vi "Get BLISS_Select Random Image.vi"(7 "BLISS Type":enum16{"Reject Images", "PBQA Images"}(ring), 8 "error in":errorcluster, 11 "Data Parameters in":T1={"Start Time"=timestamp(3690155740.033191 s since 1904-01-01), "Save to Folder"=path "", "Forces in Theater"=[{"Force Commander"="BlissUT124", "Units"=[]}, {"Force Commander"="BlissMP146", "Units"=[]}, {"Force Commander"="BlissMP145", "Units"=[]}, {"Force Commander"="BlissMP140", "Units"=[]}, {"Force Commander"="BlissMP137", "Units"=[]}, {"Force Commander"="BlissMP135", "Units"=[]}, {"Force Commander"="BlissMP134", "Units"=[]}, {"Force Commander"="BlissMP132", "Units"=[]}, {"Force Commander"="BlissMA109", "Units"=[]}, {"Force Commander"="BlissMA107", "Units"=[]}, {"Force Commander"="BlissMA106", "Units"=[]}, {"Force Commander"="BlissMA101", "Units"=[]}, {"Force Commander"="BlissLU118", "Units"=[]}, {"Force Commander"="BlissLU117", "Units"=[]}, {"Force Commander"="BlissLU116", "Units"=[]}, {"Force Commander"="BlissLU115", "Units"=[]}, {"Force Commander"="BlissLU114", "Units"=[]}, {"Force Commander"="BlissLU113", "Units"=[]}, {"Force Commander"="BlissLU111", "Units"=[]}, {"Force Commander"="BlissLL185", "Units"=[]}, {"Force Commander"="BlissLL183", "Units"=[]}, {"Force Commander"="BlissLL173", "Units"=[]}, {"Force Commander"="BlissLL172", "Units"=[]}, {"Force Commander"="BlissLL171", "Units"=[]}, {"Force Commander"="BlissJH103", "Units"=[]}, {"Force Commander"="BlissJH102", "Units"=[]}, {"Force Commander"="BlissJH101", "Units"=[]}, {"Force Commander"="BlissJE116", "Units"=[]}, {"Force Commander"="BlissJE115", "Units"=[]}, {"Force Commander"="BlissJE114", "Units"=[]}, {"Force Commander"="BlissJE111", "Units"=[]}, {"Force Commander"="BlissHD183", "Units"=[]}, {"Force Commander"="BlissHD182", "Units"=[]}, {"Force Commander"="BlissHD181", "Units"=[]}, {"Force Commander"="BlissGPDFFPL", "Units"=[]}, {"Force Commander"="BlissEUWIPES", "Units"=[]}, {"Force Commander"="BlissEU179", "Units"=[]}, {"Force Commander"="BlissEU178", "Units"=[]}, {"Force Commander"="BlissEU177", "Units"=[]}, {"Force Commander"="Blissdvds02", "Units"=[]}, {"Force Commander"="BlissDOWIPES", "Units"=[]}, {"Force Commander"="BlissCR022", "Units"=[]}, {"Force Commander"="BlissCR021", "Units"=[]}, {"Force Commander"="BlissCG167", "Units"=[]}, {"Force Commander"="BlissCG166", "Units"=[]}, {"Force Commander"="BlissCG161", "Units"=[]}, {"Force Commander"="BlissCG160", "Units"=[]}, {"Force Commander"="BlissCG159", "Units"=[]}, {"Force Commander"="BlissCG158", "Units"=[]}, {"Force Commander"="BlissCG157", "Units"=[]}, {"Force Commander"="BlissCG156", "Units"=[]}, {"Force Commander"="BlissCG151", "Units"=[]}, {"Force Commander"="BlissCB172", "Units"=[]}, {"Force Commander"="BlissCB171", "Units"=[]}, {"Force Commander"="BlissCB108", "Units"=[]}, {"Force Commander"="BlissCB107", "Units"=[]}, {"Force Commander"="BlissBV181", "Units"=[]}, {"Force Commander"="BlissBV162", "Units"=[]}, {"Force Commander"="BlissAK177", "Units"=[]}, {"Force Commander"="BlissAK176", "Units"=[]}, {"Force Commander"="BlissAK175", "Units"=[]}, {"Force Commander"="BlissAK174", "Units"=[]}, {"Force Commander"="BlissAK173", "Units"=[]}, {"Force Commander"="BlissAK172", "Units"=[]}, {"Force Commander"="BlissAK171", "Units"=[]}, {"Force Commander"="BlissAK139", "Units"=[]}, {"Force Commander"="BlissAK134", "Units"=[]}, {"Force Commander"="BlissAK131", "Units"=[]}, {"Force Commander"="BlissAH163", "Units"=[]}, {"Force Commander"="BlissAH162", "Units"=[]}, {"Force Commander"="BlissAH161", "Units"=[]}, {"Force Commander"="BlissAH122", "Units"=[]}, {"Force Commander"="BlissAH121", "Units"=[]}, {"Force Commander"="BlissAD106", "Units"=[]}, {"Force Commander"="BlissAD104", "Units"=[]}, {"Force Commander"="BlissAB105", "Units"=[]}, {"Force Commander"="BlissAB104", "Units"=[]}]}) -> (0 "error out":errorcluster, 3 "Data Parameters out":T1={"Start Time"=timestamp(3690155740.033191 s since 1904-01-01), "Save to Folder"=path "D:/One Drive PG/Procter and Gamble/Varghese, Jacob - Deep Learning Vision System/Front Ear Foldover/BLISS Rejects (only R325 + R326) - not reviewed", "Forces in Theater"=[{"Force Commander"="BlissUT124", "Units"=[]}, {"Force Commander"="BlissMP146", "Units"=[]}, {"Force Commander"="BlissMP145", "Units"=[]}, {"Force Commander"="BlissMP140", "Units"=[]}, {"Force Commander"="BlissMP137", "Units"=[]}, {"Force Commander"="BlissMP135", "Units"=[]}, {"Force Commander"="BlissMP134", "Units"=[]}, {"Force Commander"="BlissMP132", "Units"=[]}, {"Force Commander"="BlissMA109", "Units"=[]}, {"Force Commander"="BlissMA107", "Units"=[]}, {"Force Commander"="BlissMA106", "Units"=[]}, {"Force Commander"="BlissMA101", "Units"=[]}, {"Force Commander"="BlissLU118", "Units"=[]}, {"Force Commander"="BlissLU117", "Units"=[]}, {"Force Commander"="BlissLU116", "Units"=[]}, {"Force Commander"="BlissLU115", "Units"=[]}, {"Force Commander"="BlissLU114", "Units"=[]}, {"Force Commander"="BlissLU113", "Units"=[]}, {"Force Commander"="BlissLU111", "Units"=[]}, {"Force Commander"="BlissLL185", "Units"=[]}, {"Force Commander"="BlissLL183", "Units"=[]}, {"Force Commander"="BlissLL173", "Units"=[]}, {"Force Commander"="BlissLL172", "Units"=[]}, {"Force Commander"="BlissLL171", "Units"=[]}, {"Force Commander"="BlissJH103", "Units"=[]}, {"Force Commander"="BlissJH102", "Units"=[]}, {"Force Commander"="BlissJH101", "Units"=[]}, {"Force Commander"="BlissJE116", "Units"=[]}, {"Force Commander"="BlissJE115", "Units"=[]}, {"Force Commander"="BlissJE114", "Units"=[]}, {"Force Commander"="BlissJE111", "Units"=[]}, {"Force Commander"="BlissHD183", "Units"=[]}, {"Force Commander"="BlissHD182", "Units"=[]}, {"Force Commander"="BlissHD181", "Units"=[]}, {"Force Commander"="BlissGPDFFPL", "Units"=[]}, {"Force Commander"="BlissEUWIPES", "Units"=[]}, {"Force Commander"="BlissEU179", "Units"=[]}, {"Force Commander"="BlissEU178", "Units"=[]}, {"Force Commander"="BlissEU177", "Units"=[]}, {"Force Commander"="Blissdvds02", "Units"=[]}, {"Force Commander"="BlissDOWIPES", "Units"=[]}, {"Force Commander"="BlissCR022", "Units"=[]}, {"Force Commander"="BlissCR021", "Units"=[]}, {"Force Commander"="BlissCG167", "Units"=[]}, {"Force Commander"="BlissCG166", "Units"=[]}, {"Force Commander"="BlissCG161", "Units"=[]}, {"Force Commander"="BlissCG160", "Units"=[]}, {"Force Commander"="BlissCG159", "Units"=[]}, {"Force Commander"="BlissCG158", "Units"=[]}, {"Force Commander"="BlissCG157", "Units"=[]}, {"Force Commander"="BlissCG156", "Units"=[]}, {"Force Commander"="BlissCG151", "Units"=[]}, {"Force Commander"="BlissCB172", "Units"=[]}, {"Force Commander"="BlissCB171", "Units"=[]}, {"Force Commander"="BlissCB108", "Units"=[]}, {"Force Commander"="BlissCB107", "Units"=[]}, {"Force Commander"="BlissBV181", "Units"=[]}, {"Force Commander"="BlissBV162", "Units"=[]}, {"Force Commander"="BlissAK177", "Units"=[]}, {"Force Commander"="BlissAK176", "Units"=[]}, {"Force Commander"="BlissAK175", "Units"=[]}, {"Force Commander"="BlissAK174", "Units"=[]}, {"Force Commander"="BlissAK173", "Units"=[]}, {"Force Commander"="BlissAK172", "Units"=[]}, {"Force Commander"="BlissAK171", "Units"=[]}, {"Force Commander"="BlissAK139", "Units"=[]}, {"Force Commander"="BlissAK134", "Units"=[]}, {"Force Commander"="BlissAK131", "Units"=[]}, {"Force Commander"="BlissAH163", "Units"=[]}, {"Force Commander"="BlissAH162", "Units"=[]}, {"Force Commander"="BlissAH161", "Units"=[]}, {"Force Commander"="BlissAH122", "Units"=[]}, {"Force Commander"="BlissAH121", "Units"=[]}, {"Force Commander"="BlissAD106", "Units"=[]}, {"Force Commander"="BlissAD104", "Units"=[]}, {"Force Commander"="BlissAB105", "Units"=[]}, {"Force Commander"="BlissAB104", "Units"=[]}]})   [LabVIEW 2020]
uses:
  MC5e Gobal_Variables.vi
  Get BLISS_Data Paramter Actions.ctl
  MC5e Squad_Info.ctl
  MC5e Unit_Status_List.ctl
  MC5e Data_Parameters.ctl
  MC5e Terrain types.ctl
  Location.ctl
  MC5e Unit.ctl
  MC5e Force.ctl
panel:
  out "Aborting":bool
  in  "Tab Control":enum32{"PBQA", "Reject"}(tab)
  out "PBQA File List":string[](array[string])
  out "Reject File List":string[](array[string])
  out "Processing":bool=TRUE
  in  "Abort Process Button":bool
  out "Searching for":enum16{"Reject Images", "PBQA Images"}(ring)
  out "Server Name":string
  out "Reject Date":string
  out "Reject View":string
  out "Reject Code":string
  out "PBQA View":string
  out "PBQA Size":string
  out "PBQA date":string
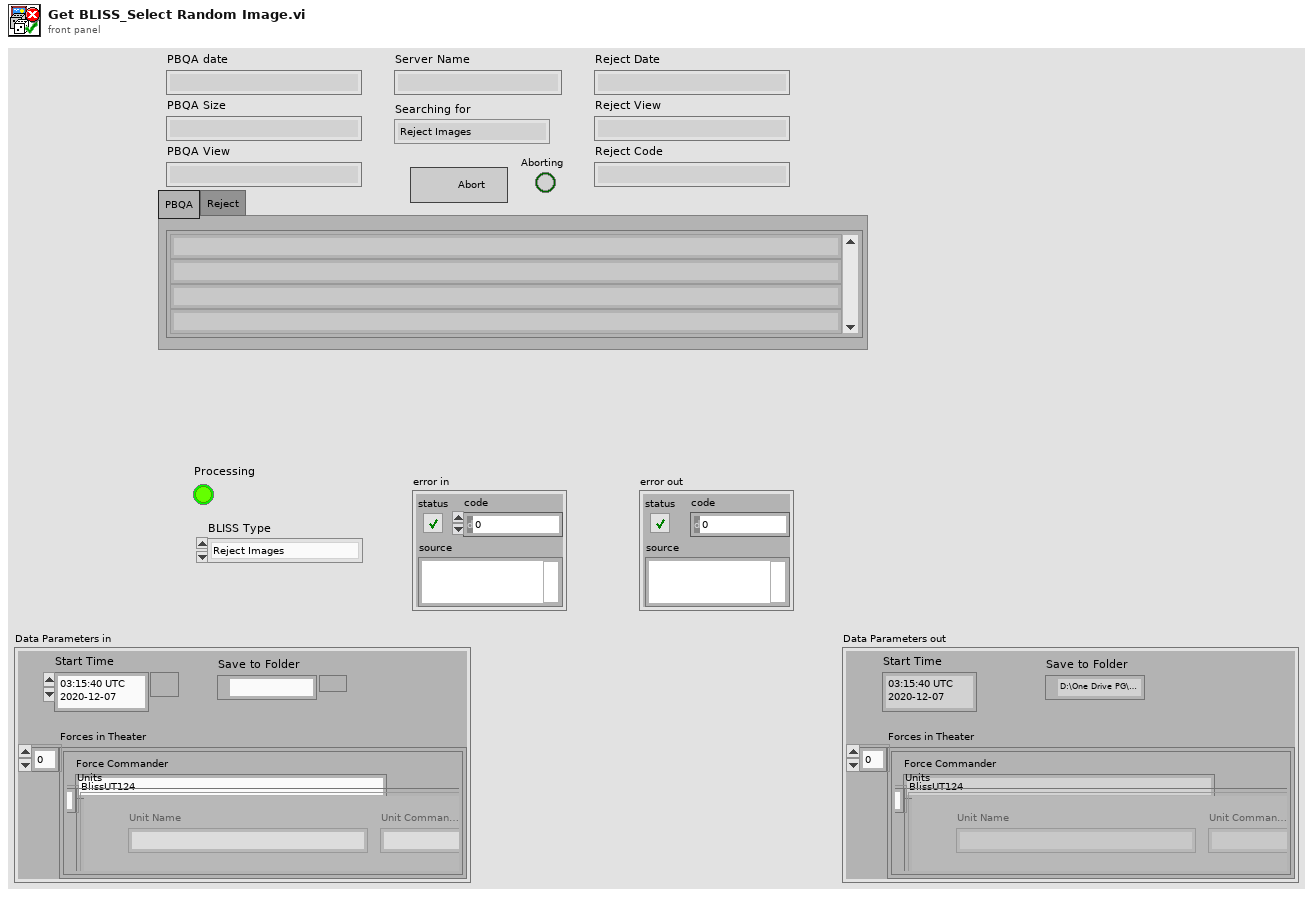
[diagram p1: front panel]
types:
  T1 = typedef "MC5e Data_Parameters.ctl" = cluster{"Start Time":timestamp, "Save to Folder":path, "Forces in Theater":T2[]}
  T2 = typedef "MC5e Force.ctl" = cluster{"Force Commander":string, "Units":T3[]}
  T3 = typedef "MC5e Unit.ctl" = cluster{"Squad List":T4, "Unit Fatigue Level":enum16{"Not Fatigued", "Fatigued", "Seriously Fatigued"}, "Flying Unit":bool, "Mounted Unit":bool, "Difficult Terrain Types":T6, "Full BR":dbl, "Defending from Stronghold":bool, "Speed":dbl, "Capacity %":dbl, "Morale":dbl, "Current BR":dbl, "Location":T7, "Unit Name":string, "Unit Commander":string, "Unit Notes":string}
  T4 = typedef "MC5e Unit_Status_List.ctl" = T5[]
  T5 = typedef "MC5e Squad_Info.ctl" = cluster{"Squad Name":string, "# Soldiers":dbl, "Battle Rating":dbl, "Flying":bool, "Mounted":bool, "Speed":dbl, "Range":dbl, "Morale":dbl, "Token Image":variant, "Max Endurance":dbl, "Current Endurance":dbl, "Difficult Terrain":T6}
  T6 = typedef "MC5e Terrain types.ctl" = cluster{"Artic / snow / ice)":bool, "Coast":bool, "Desert / sand":bool, "Forest / woodland":bool, "Grassland / plains":bool, "Mountain / canyons":bool, "Underdark / caverns":bool, "Acquatic / rivers, lakes, ocean":bool}
  T7 = typedef "Location.ctl" = cluster{"X coordinate":dbl, "Y coordinate":dbl}
  T8 = typedef "Get BLISS_Data Paramter Actions.ctl" = enum16{"Initialize", "Increment Index", "Reset Results", "Update", "Read"}
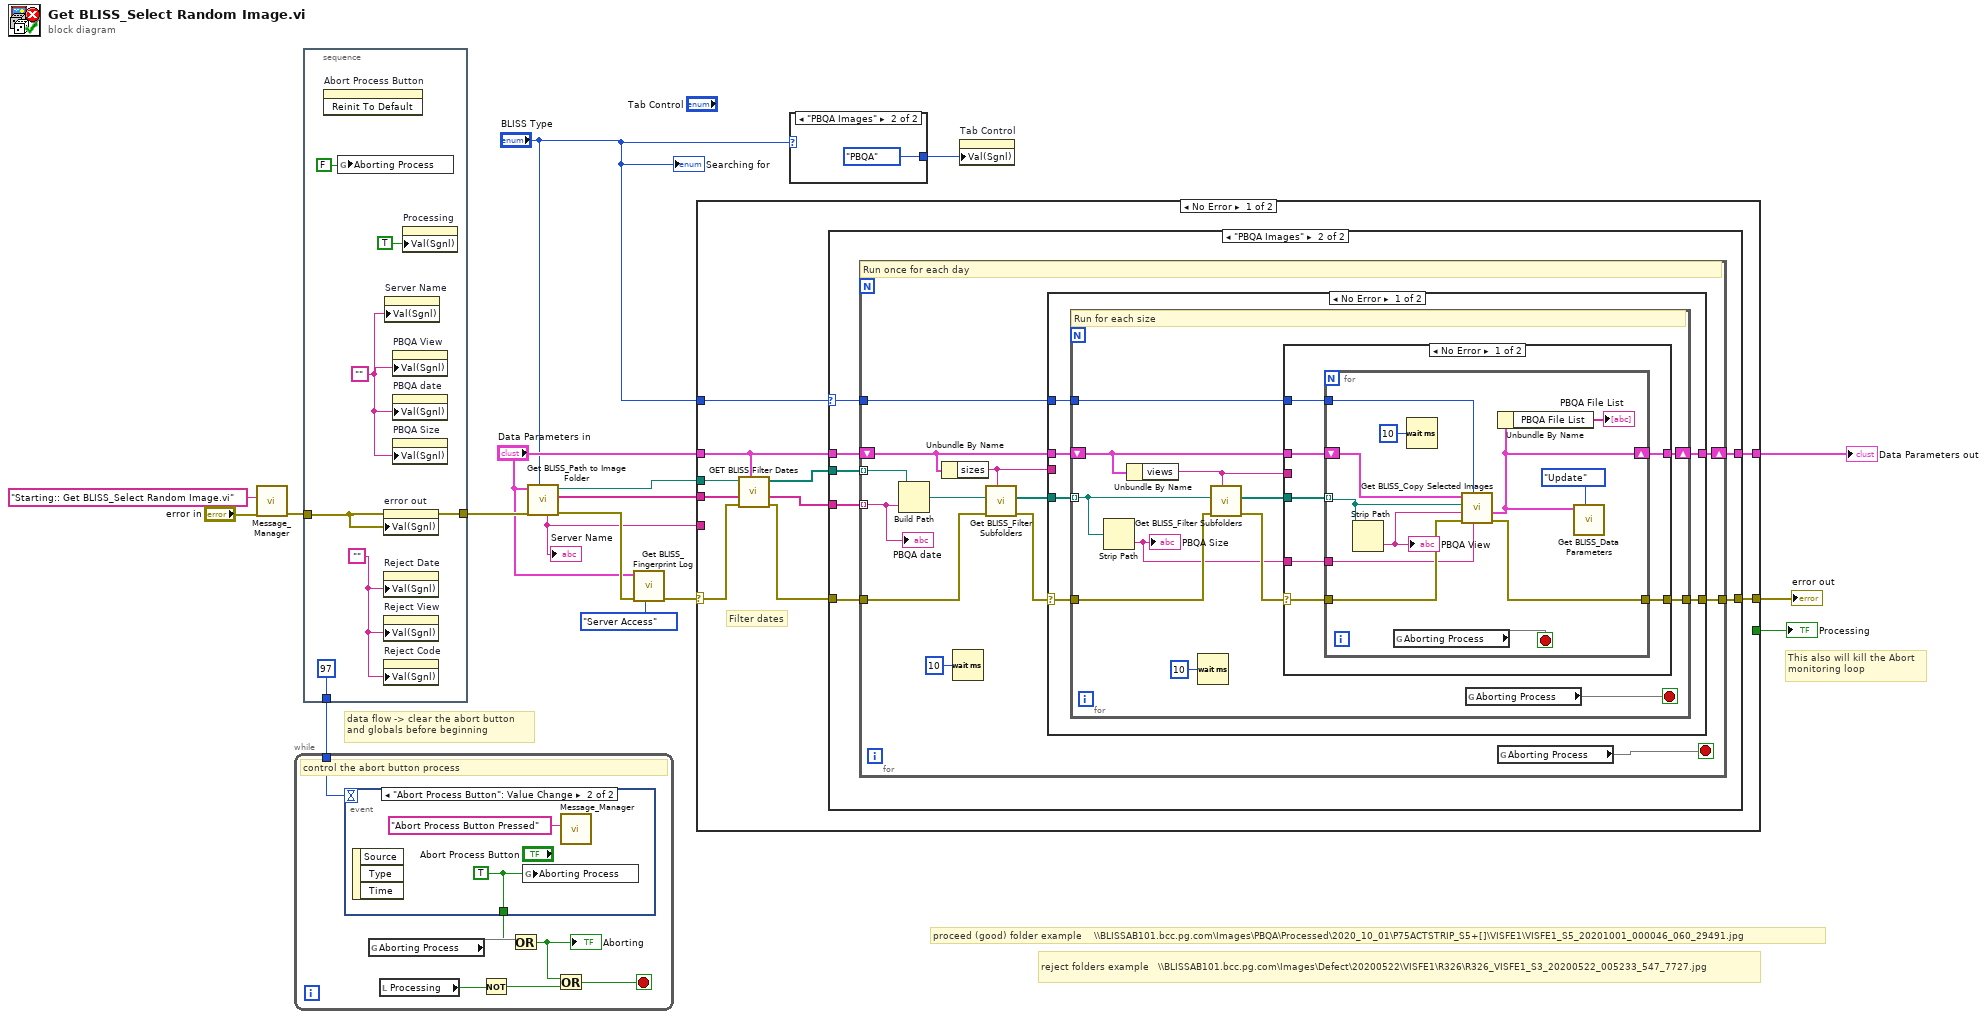
[diagram p0: block diagram]
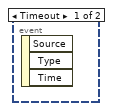
[diagram p2: hidden frame]
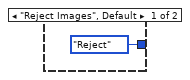
[diagram p3: hidden frame]
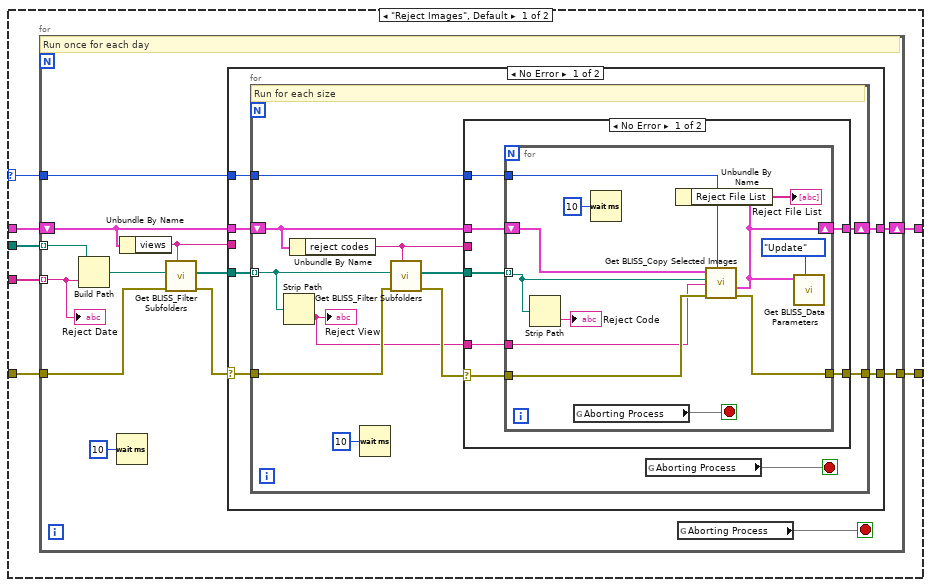
[diagram p4: hidden frame]
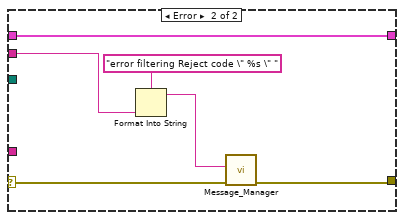
[diagram p5: hidden frame]
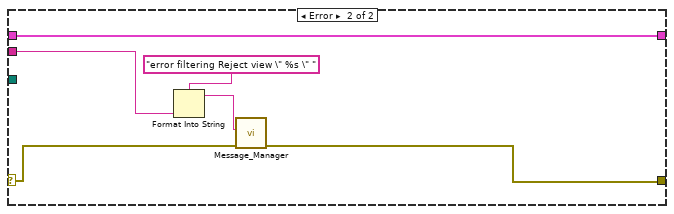
[diagram p6: hidden frame]
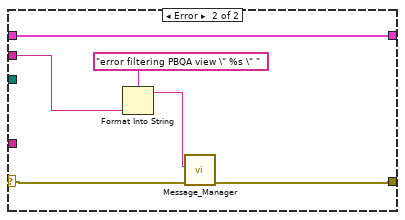
[diagram p7: hidden frame]
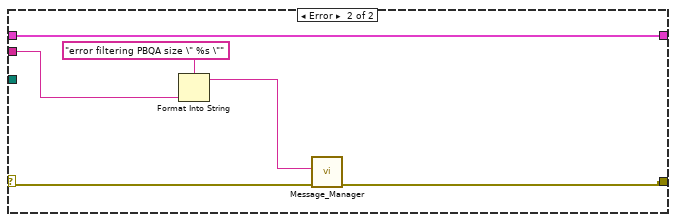
[diagram p8: hidden frame]
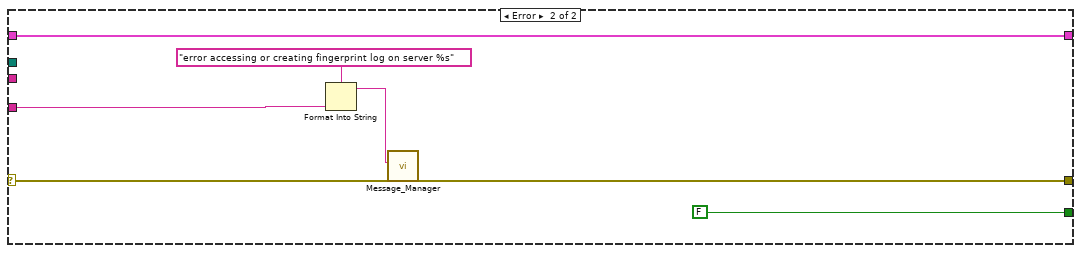
[diagram p9: hidden frame]
diagram:
  # "This also will kill the Abort\nmonitoring loop"
  # "data flow -> clear the abort button \nand globals before beginning"
  # "reject folders example   \\\\BLISSAB101.bcc.pg.com\\Images\\Defect\\20200522\\VISFE1\\R326\\R326_VISFE1_S3_20200522_005233_547_7727.jpg"
  # "proceed (good) folder example    \\\\BLISSAB101.bcc.pg.com\\Images\\PBQA\\Processed\\2020_10_01\\P75ACTSTRIP_S5+[]\\VISFE1\\VISFE1_S5_20201001_000046_060_29491.jpg"
  n1 = call "Message_Manager.vi"("error in"="error in", "New Entry"="Starting:: Get BLISS_Select Random Image.vi") -> ("error out"=w10:errorcluster)  [unwired: 4 in, 5 out]
  n2 = stacked-sequence {
    tunnel: w10 -> [w23]
    tunnel: [w22] -> w13
    tunnel: [u32 97] -> w2
    frame #0 {
      w21 = ""
      w19 = ""
      n3 = invoke on="Abort Process Button" class="Bool" method="Reinit To Default"() -> ()  [unwired: 3 in, 3 out]
      n4 = global write "MC5e Gobal_Variables.vi" "Aborting Process"(FALSE ("Value (Signaling)")) -> ()
      n5 = property on="error out" class="Clust (strict)"(error in=w23, "Val(Sgnl)"=w23) -> (error out=w22:errorcluster)  [unwired: 1 in, 1 out]
      n6 = property on="Reject Date" class="Str"("Val(Sgnl)"=w21) -> ()  [unwired: 2 in, 2 out]
      n7 = property on="Reject View" class="Str"("Val(Sgnl)"=w21) -> ()  [unwired: 2 in, 2 out]
      n8 = property on="Reject Code" class="Str"("Val(Sgnl)"=w21) -> ()  [unwired: 2 in, 2 out]
      n9 = property on="Server Name" class="Str"("Val(Sgnl)"=w19) -> ()  [unwired: 2 in, 2 out]
      n10 = property on="PBQA View" class="Str"("Val(Sgnl)"=w19) -> ()  [unwired: 2 in, 2 out]
      n11 = property on="PBQA date" class="Str"("Val(Sgnl)"=w19) -> ()  [unwired: 2 in, 2 out]
      n12 = property on="PBQA Size" class="Str"("Val(Sgnl)"=w19) -> ()  [unwired: 2 in, 2 out]
      n13 = property on="Processing" class="Bool (strict)"("Val(Sgnl)"=TRUE ("Value (Signaling)")) -> ()  [unwired: 2 in, 2 out]
    }
  }
  n14 = while {
    tunnel: w2 -> [w28]
    stop <- w29 stop-if-true
    # "control the abort button process"
    n15 = event shown="[1] \"Abort Process Button\": Value Change" {
      selector: _ -> [_ _]
      dyn-events: _ -> [_ _]
      timeout: w28 -> [_ _]
      tunnel: [_ w32] -> w26
      event Timeout {
        n16 = event-data() -> ()  [unwired: 1 in, 3 out]
      }
      event "Abort Process Button": Value Change {
        w32 = TRUE ("Aborting Process")
        n17 = event-data() -> ()  [unwired: 1 in, 3 out]
        n18 = global write "MC5e Gobal_Variables.vi" "Aborting Process"(w32) -> ()
        n19 = call "Message_Manager.vi"("New Entry"="Abort Process Button Pressed") -> ()  [unwired: 5 in, 6 out]
      }
    }
    n20 = global read "MC5e Gobal_Variables.vi" "Aborting Process"() -> (w27)
    n21 = local read "Processing"() -> (w31:bool)
    n22 = Not(x=w31) -> (.not. x?=w30:bool)
    n23 = Or(x=w26, y=w27) -> (x .or. y?=w25:bool)
    "Aborting" <- w25
    n24 = Or(x=w25, y=w30) -> (x .or. y?=w29:bool)
  }
  n25 = call "Get BLISS_Path to Image Folder.vi"("BLISS Type"="BLISS Type", "error in (no error)"=w13, "Data Parameters in"="Data Parameters in") -> ("error out"=w8:errorcluster, "Dates (folders)"=w16:string[], "Server Images Path"=w17:path, "Server Name"=w7:string)  [unwired: 5 in]
  "Server Name" <- w7
  n26 = call "Get BLISS_Fingerprint Log.vi"("Action"=enum16{"Server Access", "File Access"}."Server Access", "error in (no error)"=w8, "Data Parameters in"="Data Parameters in") -> ("error out"=w1:errorcluster)  [unwired: 8 in]
  n27 = case shown="No Error" w1 {
    selector: w1 -> [w37 w187]
    tunnel: w16 -> [w39 _]
    tunnel: w17 -> [w40 _]
    tunnel: [w43 w187] -> w15
    tunnel: "Data Parameters in" -> [w34 w186]
    tunnel: [w42 w186] -> w9
    tunnel: "BLISS Type" -> [w41 _]
    tunnel: [_ FALSE] -> w14
    tunnel: w7 -> [_ w182]
    frame No Error {
      # "Filter dates"
      n28 = call "GET BLISS Filter Dates.vi"("Data Parameters in"=w34, "error in"=w37, "Dates (folders)"=w39, "Server Images Path"=w40) -> ("error out"=w36:errorcluster, "Valid Dates"=w35:string[], "Valid Paths"=w38:path[])  [unwired: 5 in]
      n29 = case shown="\"PBQA Images\"" w41 {
        selector: w41 -> [w44 w113]
        tunnel: w38 -> [w50 w119]
        tunnel: w35 -> [w49 w118]
        tunnel: [w48 w117] -> w43
        tunnel: w34 -> [w47 w116]
        tunnel: w36 -> [w46 w115]
        tunnel: [w45 w114] -> w42
        frame "Reject Images", Default {
          n30 = for {
            tunnel: w50 -> [w63] mode=indexing
            tunnel: w49 -> [w61] mode=indexing
            shift-right: [w60] -> w45
            shift-left: w47 -> [w59]
            tunnel: w44 -> [w54]
            tunnel: w46 -> [w56]
            tunnel: [w62] -> w48
            stop <- w53 stop-if-true
            # "Run once for each day"
            n31 = Build Path(base path=w63, name or relative path=w61) -> (appended path=w58:path)
            n32 = Wait (ms)(milliseconds to wait=u32 10) -> ()  [unwired: 1 out]
            n33 = Unbundle By Name(w59) -> ("views"=w51:string)
            n34 = call "Get BLISS_Filter Subfolders.vi"("Folder Criteria\n(comma delimited)"=w51, "error in"=w56, "parent path"=w58) -> ("error out"=w55:errorcluster, "Valid Paths"=w57:path[])  [unwired: 7 in]
            n35 = case shown="No Error" w55 {
              selector: w55 -> [w66 w111]
              tunnel: [w69 w107] -> w62
              tunnel: w59 -> [w68 w112]
              tunnel: [w67 w112] -> w60
              tunnel: w57 -> [w65 _]
              tunnel: w54 -> [w64 _]
              tunnel: w51 -> [_ w108]
              frame No Error {
                n36 = for {
                  shift-right: [w80] -> w67
                  shift-left: w68 -> [w79]
                  tunnel: w65 -> [w78] mode=indexing
                  tunnel: w64 -> [w74]
                  tunnel: w66 -> [w77]
                  tunnel: [w81] -> w69
                  stop <- w73 stop-if-true
                  # "Run for each size"
                  n37 = Strip Path(path=w78) -> (name=w71:string)  [unwired: 1 out]
                  "Reject View" <- w71
                  n38 = Unbundle By Name(w79) -> ("reject codes"=w70:string)
                  n39 = Wait (ms)(milliseconds to wait=u32 10) -> ()  [unwired: 1 out]
                  n40 = call "Get BLISS_Filter Subfolders.vi"("Folder Criteria\n(comma delimited)"=w70, "error in"=w77, "parent path"=w78) -> ("error out"=w76:errorcluster, "Valid Paths"=w75:path[])  [unwired: 7 in]
                  n41 = case shown="No Error" w76 {
                    selector: w76 -> [w85 w105]
                    tunnel: [w88 w104] -> w81
                    tunnel: w79 -> [w87 w106]
                    tunnel: [w86 w106] -> w80
                    tunnel: w75 -> [w84 _]
                    tunnel: w74 -> [w83 _]
                    tunnel: w71 -> [w82 _]
                    tunnel: w70 -> [_ w102]
                    frame No Error {
                      n42 = for {
                        shift-right: [w89] -> w86
                        shift-left: w87 -> [w97]
                        tunnel: w84 -> [w98] mode=indexing
                        tunnel: w83 -> [w96]
                        tunnel: w85 -> [w100]
                        tunnel: [w93] -> w88
                        tunnel: w82 -> [w91]
                        stop <- w94 stop-if-true
                        n43 = Strip Path(path=w98) -> (name=→"Reject Code":string)  [unwired: 1 out]
                        n44 = global read "MC5e Gobal_Variables.vi" "Aborting Process"() -> (w94)
                        n45 = Wait (ms)(milliseconds to wait=u32 10) -> ()  [unwired: 1 out]
                        n46 = call "Get BLISS_Copy Selected Images.vi"("BLISS Type"=w96, "error in (no error)"=w100, "View"=w91, "base path"=w98, "Data Parameters in"=w97) -> ("error out"=w93:errorcluster, "Data Parameters Out"=w89:T1)  [unwired: 5 in]
                        n47 = Unbundle By Name(w89) -> ("Reject File List"=→"Reject File List":string[])
                        n48 = call "Get BLISS_Data Parameters.vi"("Data Action (Read)"=Get_BLISS_Data_Paramter_Actions."Update", "Data Parameters in"=w89) -> ()  [unwired: 7 in, 3 out]
                      }
                    }
                    frame Error {
                      n49 = Format Into String(format string="error filtering Reject code \" %s \" " ("New Entry"), w102) -> (resulting string=w101:string)  [unwired: 2 in, 1 out]
                      n50 = call "Message_Manager.vi"("error in"=w105, "New Entry"=w101) -> ("error out"=w104:errorcluster)  [unwired: 4 in, 5 out]
                    }
                  }
                  n51 = global read "MC5e Gobal_Variables.vi" "Aborting Process"() -> (w73)
                }
              }
              frame Error {
                n52 = Format Into String(format string="error filtering Reject view \" %s \" " ("New Entry"), w108) -> (resulting string=w109:string)  [unwired: 2 in, 1 out]
                n53 = call "Message_Manager.vi"("error in"=w111, "New Entry"=w109) -> ("error out"=w107:errorcluster)  [unwired: 4 in, 5 out]
              }
            }
            n54 = global read "MC5e Gobal_Variables.vi" "Aborting Process"() -> (w53)
            "Reject Date" <- w61
          }
        }
        frame "PBQA Images" {
          n55 = for {
            tunnel: w119 -> [w132] mode=indexing
            tunnel: w118 -> [w130] mode=indexing
            shift-right: [w129] -> w114
            shift-left: w116 -> [w128]
            tunnel: w113 -> [w123]
            tunnel: w115 -> [w125]
            tunnel: [w131] -> w117
            stop <- w122 stop-if-true
            # "Run once for each day"
            n56 = Build Path(base path=w132, name or relative path=w130) -> (appended path=w127:path)
            n57 = Unbundle By Name(w128) -> ("sizes"=w120:string)
            n58 = Wait (ms)(milliseconds to wait=u32 10) -> ()  [unwired: 1 out]
            n59 = call "Get BLISS_Filter Subfolders.vi"("Folder Criteria\n(comma delimited)"=w120, "error in"=w125, "parent path"=w127) -> ("error out"=w124:errorcluster, "Valid Paths"=w126:path[])  [unwired: 7 in]
            n60 = case shown="No Error" w124 {
              selector: w124 -> [w135 w180]
              tunnel: [w138 w179] -> w131
              tunnel: w128 -> [w137 w181]
              tunnel: [w136 w181] -> w129
              tunnel: w126 -> [w134 _]
              tunnel: w123 -> [w133 _]
              tunnel: w120 -> [_ w177]
              frame No Error {
                n61 = for {
                  shift-right: [w149] -> w136
                  shift-left: w137 -> [w148]
                  tunnel: w134 -> [w147] mode=indexing
                  tunnel: w133 -> [w143]
                  tunnel: w135 -> [w146]
                  tunnel: [w150] -> w138
                  stop <- w142 stop-if-true
                  # "Run for each size"
                  n62 = Strip Path(path=w147) -> (name=w139:string)  [unwired: 1 out]
                  "PBQA Size" <- w139
                  n63 = Unbundle By Name(w148) -> ("views"=w140:string)
                  n64 = Wait (ms)(milliseconds to wait=u32 10) -> ()  [unwired: 1 out]
                  n65 = call "Get BLISS_Filter Subfolders.vi"("Folder Criteria\n(comma delimited)"=w140, "error in"=w146, "parent path"=w147) -> ("error out"=w145:errorcluster, "Valid Paths"=w144:path[])  [unwired: 7 in]
                  n66 = case shown="No Error" w145 {
                    selector: w145 -> [w154 w174]
                    tunnel: [w157 w173] -> w150
                    tunnel: w148 -> [w156 w175]
                    tunnel: [w155 w175] -> w149
                    tunnel: w144 -> [w153 _]
                    tunnel: w143 -> [w152 _]
                    tunnel: w140 -> [_ w171]
                    tunnel: w139 -> [w151 _]
                    frame No Error {
                      n67 = for {
                        shift-right: [w159] -> w155
                        shift-left: w156 -> [w167]
                        tunnel: w153 -> [w168] mode=indexing
                        tunnel: w152 -> [w166]
                        tunnel: w154 -> [w169]
                        tunnel: [w163] -> w157
                        tunnel: w151 -> [w158]
                        stop <- w164 stop-if-true
                        n68 = Strip Path(path=w168) -> (name=w161:string)  [unwired: 1 out]
                        "PBQA View" <- w161
                        n69 = global read "MC5e Gobal_Variables.vi" "Aborting Process"() -> (w164)
                        n70 = Wait (ms)(milliseconds to wait=u32 10) -> ()  [unwired: 1 out]
                        n71 = call "Get BLISS_Copy Selected Images.vi"("Size"=w158, "BLISS Type"=w166, "error in (no error)"=w169, "View"=w161, "base path"=w168, "Data Parameters in"=w167) -> ("error out"=w163:errorcluster, "Data Parameters Out"=w159:T1)  [unwired: 4 in]
                        n72 = Unbundle By Name(w159) -> ("PBQA File List"=→"PBQA File List":string[])
                        n73 = call "Get BLISS_Data Parameters.vi"("Data Action (Read)"=Get_BLISS_Data_Paramter_Actions."Update", "Data Parameters in"=w159) -> ()  [unwired: 7 in, 3 out]
                      }
                    }
                    frame Error {
                      n74 = Format Into String(format string="error filtering PBQA view \" %s \" " ("New Entry"), w171) -> (resulting string=w170:string)  [unwired: 2 in, 1 out]
                      n75 = call "Message_Manager.vi"("error in"=w174, "New Entry"=w170) -> ("error out"=w173:errorcluster)  [unwired: 4 in, 5 out]
                    }
                  }
                  n76 = global read "MC5e Gobal_Variables.vi" "Aborting Process"() -> (w142)
                }
              }
              frame Error {
                n77 = Format Into String(format string="error filtering PBQA size \" %s \"" ("New Entry"), w177) -> (resulting string=w176:string)  [unwired: 2 in, 1 out]
                n78 = call "Message_Manager.vi"("error in"=w180, "New Entry"=w176) -> ("error out"=w179:errorcluster)  [unwired: 4 in, 5 out]
              }
            }
            n79 = global read "MC5e Gobal_Variables.vi" "Aborting Process"() -> (w122)
            "PBQA date" <- w130
          }
        }
      }
    }
    frame Error {
      n80 = Format Into String(format string="error accessing or creating fingerprint log on server %s" ("New Entry"), w182) -> (resulting string=w183:string)  [unwired: 2 in, 1 out]
      n81 = call "Message_Manager.vi"("New Entry"=w183) -> ()  [unwired: 5 in, 6 out]
    }
  }
  "error out" <- w15
  "Processing" <- w14
  "Data Parameters out" <- w9
  n82 = case shown="\"PBQA Images\"" "BLISS Type" {
    tunnel: [enum32{"PBQA", "Reject"}."Reject" ("Value (Signaling)") enum32{"PBQA", "Reject"}."PBQA" ("Value (Signaling)")] -> w4
    frame "Reject Images", Default {
    }
    frame "PBQA Images" {
    }
  }
  n83 = property on="Tab Control" class="TabCtl (strict)"("Val(Sgnl)"=w4) -> ()  [unwired: 2 in, 2 out]
  "Searching for" <- "BLISS Type"
